vi "JAC_L_InputPort_FGV.vi"(8 "Error In":errorcluster, 10 "LPO Status Set":bool[](array[boolean]), 11 "Enum":enum16{"1. LPO_Input Read", "2. LPO_Input Set"}(ring)) -> (0 "Error Out":errorcluster, 2 "LPO Status Read":bool[](array[boolean]))   [LabVIEW 2015]
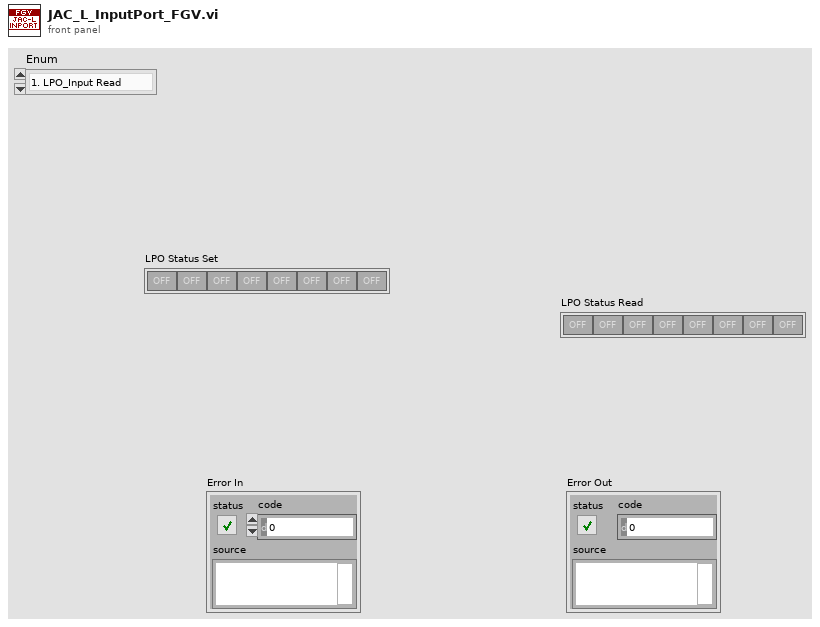
[diagram p1: front panel]
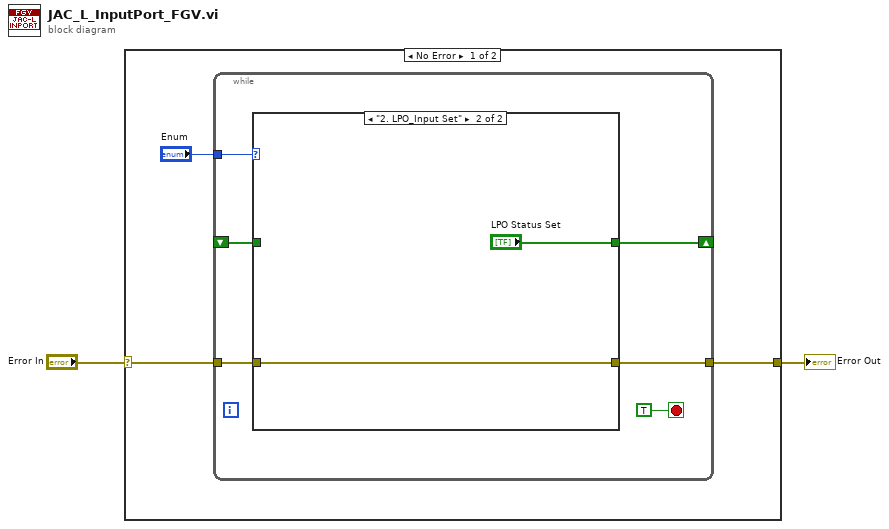
[diagram p0: block diagram]
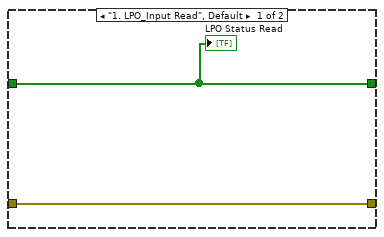
[diagram p2: hidden frame]
diagram:
  n1 = case shown="No Error" "Error In" {
    selector: "Error In" -> [w4 w16]
    tunnel: [w3 w16] -> w1
    frame No Error {
      n2 = while {
        tunnel: "Enum" -> [w11]
        shift-right: [w9] -> _
        shift-left: _ -> [w8]
        tunnel: w4 -> [w7]
        tunnel: [w6] -> w3
        stop <- TRUE stop-if-true
        n3 = case shown="\"2. LPO_Input Set\"" w11 {
          tunnel: [w12 "LPO Status Set"] -> w9
          tunnel: w8 -> [w12 _]
          tunnel: w7 -> [w13 w15]
          tunnel: [w13 w15] -> w6
          frame "1. LPO_Input Read", Default {
            "LPO Status Read" <- w12
          }
          frame "2. LPO_Input Set" {
          }
        }
      }
    }
    frame Error {
    }
  }
  "Error Out" <- w1
